vi "libssh2_channel_write_ex.vi"(8 "error in (no error)":errorcluster, 9 "buffer":u8[](array[numeric]), 10 "stream id":i32, 11 "channel":T1) -> (0 "error out":errorcluster, 3 "bytes written":i32)   [LabVIEW 2013, in "libssh2.lvlib"]
doc: "Write data to a channel."
uses:
  libssh2.lvlib
  Channel Refnum.ctl
  Acquire Session.vi
  Release Session.vi
  Not A Channel.vi
  <vilib>/Utility/error.llb/Error Cluster From Error Code.vi
  Global Settings.vi
  Read Channel Refnum.vi
  Read Session Refnum.vi
  <vilib>/Utility/semaphor.llb/Acquire Semaphore.vi
  <vilib>/Utility/semaphor.llb/Release Semaphore.vi
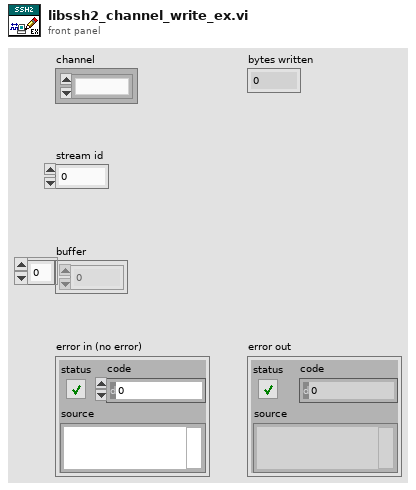
[diagram p1: front panel]
types:
  T1 = typedef "libssh2.lvlib/Channel Refnum.ctl" = refnum<k1>
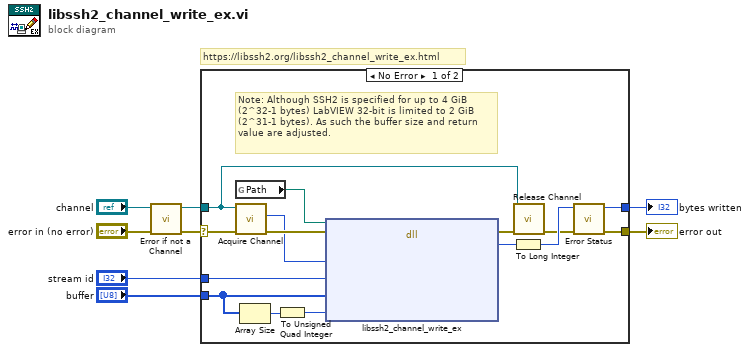
[diagram p0: block diagram]
diagram:
  # "https://libssh2.org/libssh2_channel_write_ex.html"
  n1 = call "Error if not a Channel.vi"("error in (no error)"="error in (no error)", "channel"="channel") -> ("error out"=w3:errorcluster, "channel out"=w1:T1)  [unwired: 8 in]
  n2 = case shown="No Error" w3 {
    selector: w3 -> [w21 w24]
    tunnel: [w20 w24] -> w8
    tunnel: "stream id" -> [w23 _]
    tunnel: "buffer" -> [w22 _]
    tunnel: [w19 _] -> w5
    tunnel: w1 -> [w9 _]
    frame No Error {
      # "Note: Although SSH2 is specified for up to 4 GiB\n(2^32-1 bytes) LabVIEW 32-bit is limited to 2 GiB\n(2^31-1 bytes). As such the buffer size and return\nvalue are adjusted."
      n3 = global read "Global Settings.vi" "Path"() -> (w13:path)
      n4 = call "Acquire Channel.vi"("error in (no error)"=w21, "channel"=w9) -> ("error out"=w15:errorcluster, "LIBSSH2_CHANNEL*"=w14:u64)  [unwired: 8 in]
      n5 = Array Size(array=w22) -> (size(s)=w17:i32)
      n6 = To Unsigned Quad Integer(1:w17) -> (0:w16:u64)
      n7 = dll-call lib="?" fn="libssh2_channel_write_ex"(path in=w13, error in=w15, "channel"=w14, "stream_id"=w23, "buf"=w22, "buflen"=w16) -> (error out=w18:errorcluster, "return value"=w12:i64)  [unwired: 5 in, 1 out]
      n8 = To Long Integer(number=w12) -> (32bit integer=w11:i32)
      n9 = call "Release Channel.vi"("error in (no error)"=w18, "channel"=w9) -> ("error out"=w10:errorcluster)  [unwired: 9 in]
      n10 = call "Error Status.vi"("error in (no error)"=w10, "return value"=w11) -> ("error out"=w20:errorcluster, "return value out"=w19:i32)  [unwired: 8 in]
    }
    frame Error {
    }
  }
  "error out" <- w8
  "bytes written" <- w5
